vi "Test.vi"(11 "info":string[](array[string])=["Signal Mean", "12.00", "Signal RMS", "10.1"]) -> ()   [LabVIEW 2014]
uses:
  E:/Files/subversion/C3/NIWeek/SepOfConcerns/Source/DotNet/ClientDialogs/ClientDialogs/bin/Debug/ClientDialogs.dll
  bin/Debug/ClientDialogs.dll
panel:
  out "error out":errorcluster
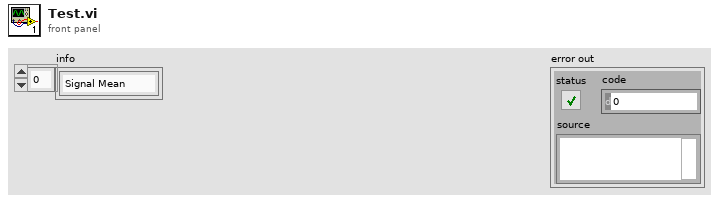
[diagram p1: front panel]
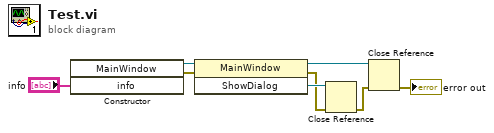
[diagram p0: block diagram]
diagram:
  n1 = constructor class="MainWindow"("info"="info") -> (reference out=w7:refnum<k24>, error out=w5:errorcluster)  [unwired: 3 in, 2 out]
  n2 = invoke class="MainWindow" method="ShowDialog"(reference=w7, error in=w5) -> (reference out=w6:refnum<k24>, error out=w2:errorcluster, "ShowDialog"=w3:refnum<k24>)  [unwired: 1 in]
  n3 = Close Reference(reference=w3, error in (no error)=w2) -> (error out=w1:errorcluster)
  n4 = Close Reference(reference=w6, error in (no error)=w1) -> (error out=→"error out":errorcluster)
